vi "Determine Warning - Temperature and Wind subVIs.vi"(6 "High Wind Speed":dbl, 7 "Current Wind Speed":dbl, 8 "error in (no error)":errorcluster, 9 "Low Temp":dbl, 10 "High Temp":dbl, 11 "Current Temperature":dbl) -> (0 "error out":errorcluster, 1 "Warning?":bool, 2 "Warning Text":string)   [LabVIEW 2010]
doc: "This VI is one solution to an exercise in the LabVIEW Core II course. In this exercise, you take inherited code and improve it for readability and maintainability."
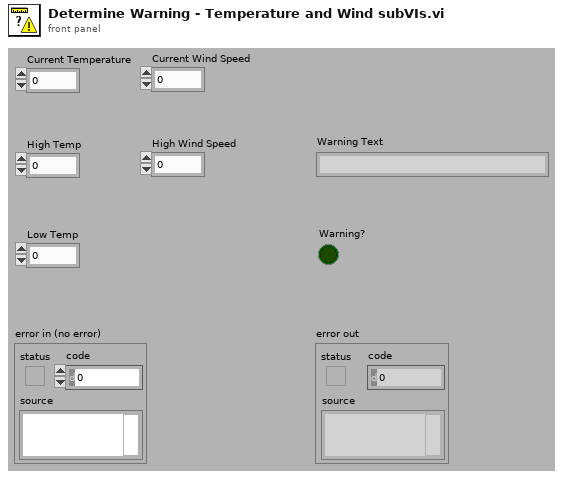
[diagram p1: front panel]
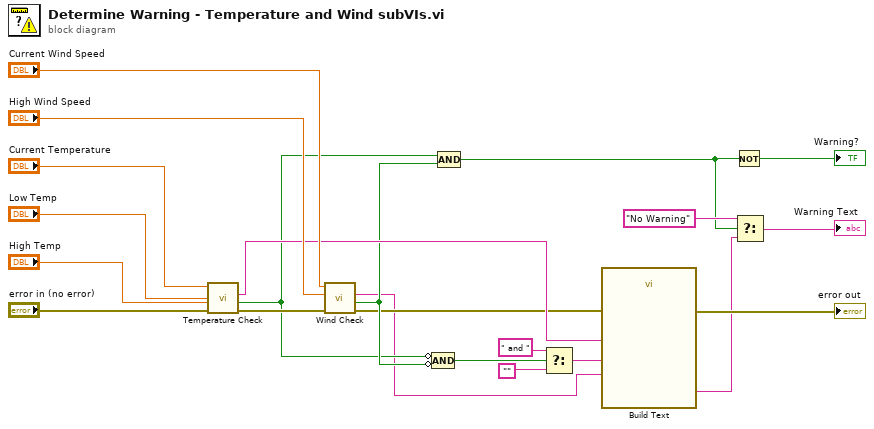
[diagram p0: block diagram]
diagram:
  n1 = call "Temperature Check.vi"("error in (no error)"="error in (no error)", "High Temp"="High Temp", "Low Temp"="Low Temp", "Current Temperature"="Current Temperature") -> ("error out"=w5:errorcluster, "Temperature Warning?"=w3:bool, "Temperature Warning"=w13:string)  [unwired: 5 out]
  n2 = call "Wind Check.vi"("error in (no error)"=w5, "High Wind Speed"="High Wind Speed", "Current Wind Speed"="Current Wind Speed") -> ("error out"=w2:errorcluster, "Wind Warning?"=w4:bool, "Wind Warning Msg"=w1:string)  [unwired: 6 out]
  n3 = Compound Arithmetic op=AND(invert w3, invert w4) -> (w7:bool)
  n4 = Compound Arithmetic op=AND(w3, w4) -> (w6:bool)
  n5 = Select(t=" and ", s=w7, f="") -> (s? t:f=w11:string)
  n6 = call "Build Text"("Temp Warning"=w13, "And"=w11, "Freeze Warning"=w1, "error in (no error)"=w2) -> ("Result"=w8:string, "error out"=→"error out":errorcluster)  [unwired: 1 in, 9 out]
  n7 = Not(x=w6) -> (.not. x?=→"Warning?":bool)
  n8 = Select(t="No Warning", s=w6, f=w8) -> (s? t:f=→"Warning Text":string)
